vi "Circle Diameters.vi"() -> ()   [LabVIEW 2020]
panel:
  out "Diametro [mm]":dbl[](array[numeric])
  out "error out":errorcluster
  out "Diametro [mm]":dbl[](array[numeric])
  in  "calibration Image":path=path "C:/Users/Dell/Documents/Vision-System/Images/calib-info_2mm.png"
  out "Image":T1(plugin-control)
  in  "error in (no error)":errorcluster
  in  "Image Path":path=path "C:/Users/Dell/Documents/Vision-System/Images/Piletta52_scura.png"
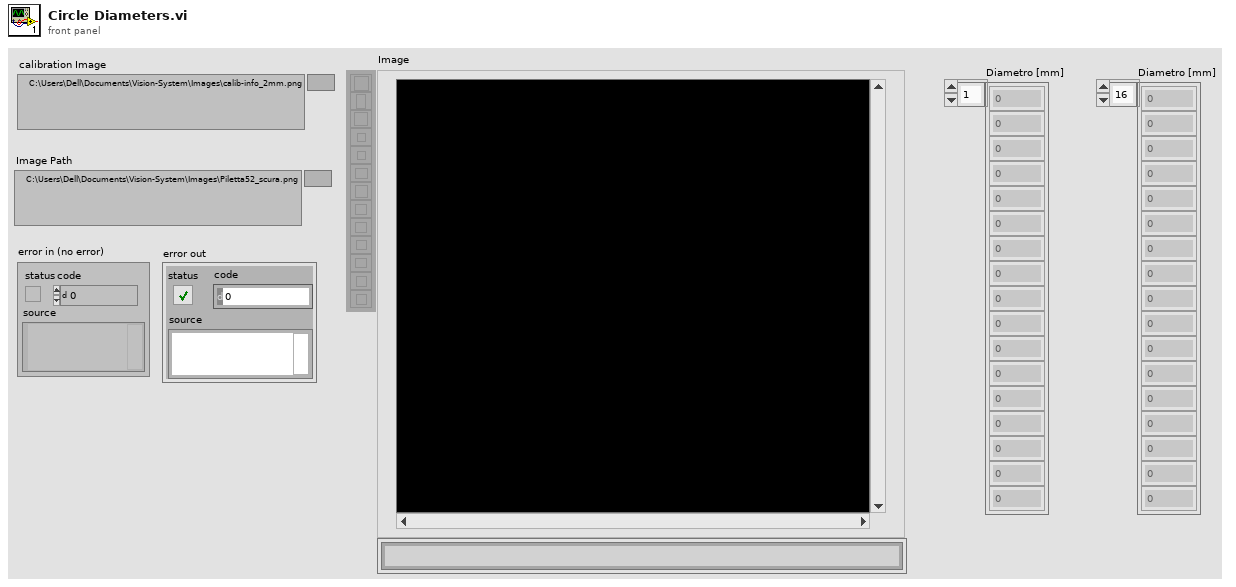
[diagram p1: front panel]
types:
  T1 = typedef "IMAQ Image.ctl" = refnum<image>
  T2 = cluster{"Center (Pixels)":cluster{"X":sgl, "Y":sgl}, "Radius (Pixels)":dbl, "Center (Real-World)":cluster{"X":sgl, "Y":sgl}, "Radius (Real-World)":dbl, "Roundness (Real-World)":dbl, "Average Strength":dbl, "Average SNR (dB)":dbl}[]
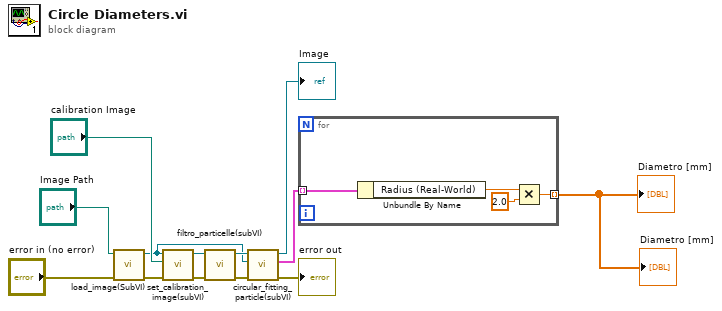
[diagram p0: block diagram]
diagram:
  n1 = call "load_image(SubVI).vi"("error in (no error)"="error in (no error)", "Image Path"="Image Path") -> ("error out"=w8:errorcluster, "Image GRAY"=w6:T1)  [unwired: 8 in]
  n2 = call "set_calibration_image(subVI).vi"("error in (no error)"=w8, "File Path"="calibration Image", "Image Dst"=w6) -> ("error out"=w9:errorcluster, "Image Out"=w10:T1)  [unwired: 6 in, 1 out]
  n3 = call "filtro_particelle(subVI).vi"("error in (no error)"=w9, "Image Src"=w10) -> ("error out"=w5:errorcluster, "Image"=w7:T1)  [unwired: 8 in]
  n4 = call "circular_fitting_particle(subVI).vi"("error in (no error)"=w5, "Image Dst"=w6, "Image Src"=w7) -> ("error out"=→"error out":errorcluster, "Array"=w3:T2, "Image Out"=→"Image":T1)  [unwired: 6 in]
  n5 = for {
    tunnel: w3 -> [w17] mode=indexing
    tunnel: [w14] -> w1 mode=indexing
    n6 = Unbundle By Name(w17) -> ("Radius (Real-World)"=w16:dbl)
    n7 = Multiply(x=w16, y=2.0) -> (x*y=w14:dbl)
  }
  "Diametro [mm]" <- w1
  "Diametro [mm]" <- w1
